vi "Is Number an IP Address.vi"(11 "UI Data in":T1={"Data Display"="", "FP Control Refs"={"Connect to Station Ref"=refnum, "Download Ref"=refnum, "Exit Button Ref"=refnum, "Start Date Refnum"=refnum, "End Date Refnum"=refnum, "Path"=refnum, "COM Port"="", "IP or Phone Ref"=refnum, "TCPIP ID"=refnum, "Reboot Refnum"=refnum, "Datafile Refnum"=refnum}, "FP Indicator Refs"={"Connected Refnum"=refnum, "Data Display Ref"=refnum, "Station ID Ref"=refnum}, "User Events"={"Stop"=refnum, "Update Display"=refnum}, "Message Queues"={"UI"=refnum, "ACQUISITION"=refnum, "PROCESSING"=refnum, "LOGGING"=refnum}, "IS IP?"=FALSE, "Downloading?"=FALSE, "DCP Version"=enum."XPert2", "Processing Loop State"=enum."Get Station  ID", "Username"=refnum, "Password"=refnum}) -> (2 "IS IP?":bool, 3 "UI Data out":T1={"Data Display"="", "FP Control Refs"={"Connect to Station Ref"=refnum, "Download Ref"=refnum, "Exit Button Ref"=refnum, "Start Date Refnum"=refnum, "End Date Refnum"=refnum, "Path"=refnum, "COM Port"="", "IP or Phone Ref"=refnum, "TCPIP ID"=refnum, "Reboot Refnum"=refnum, "Datafile Refnum"=refnum}, "FP Indicator Refs"={"Connected Refnum"=refnum, "Data Display Ref"=refnum, "Station ID Ref"=refnum}, "User Events"={"Stop"=refnum, "Update Display"=refnum}, "Message Queues"={"UI"=refnum, "ACQUISITION"=refnum, "PROCESSING"=refnum, "LOGGING"=refnum}, "IS IP?"=FALSE, "Downloading?"=FALSE, "DCP Version"=enum."XPert2", "Processing Loop State"=enum."Get Station  ID", "Username"=refnum, "Password"=refnum})   [LabVIEW 2018]
uses:
  controls/GLDL UI Data.ctl
  controls/Disconnect Control.ctl
  controls/Download Control.ctl
  controls/Exit Control.ctl
  controls/Date Control.ctl
  controls/IP Phone Number Control.ctl
  controls/Reboot Control.ctl
  controls/Connected Indicator.ctl
  controls/Output Indicator.ctl
  controls/Station ID Indicator.ctl
  Message Queue/All Message Queues.ctl
  Message Queue/Message Cluster.ctl
  controls/Processing Loop State.ctl
  Message Queue/GLDL Message Queue.lvlib
panel:
  in  "string":string
  out "IS IP? 2":bool
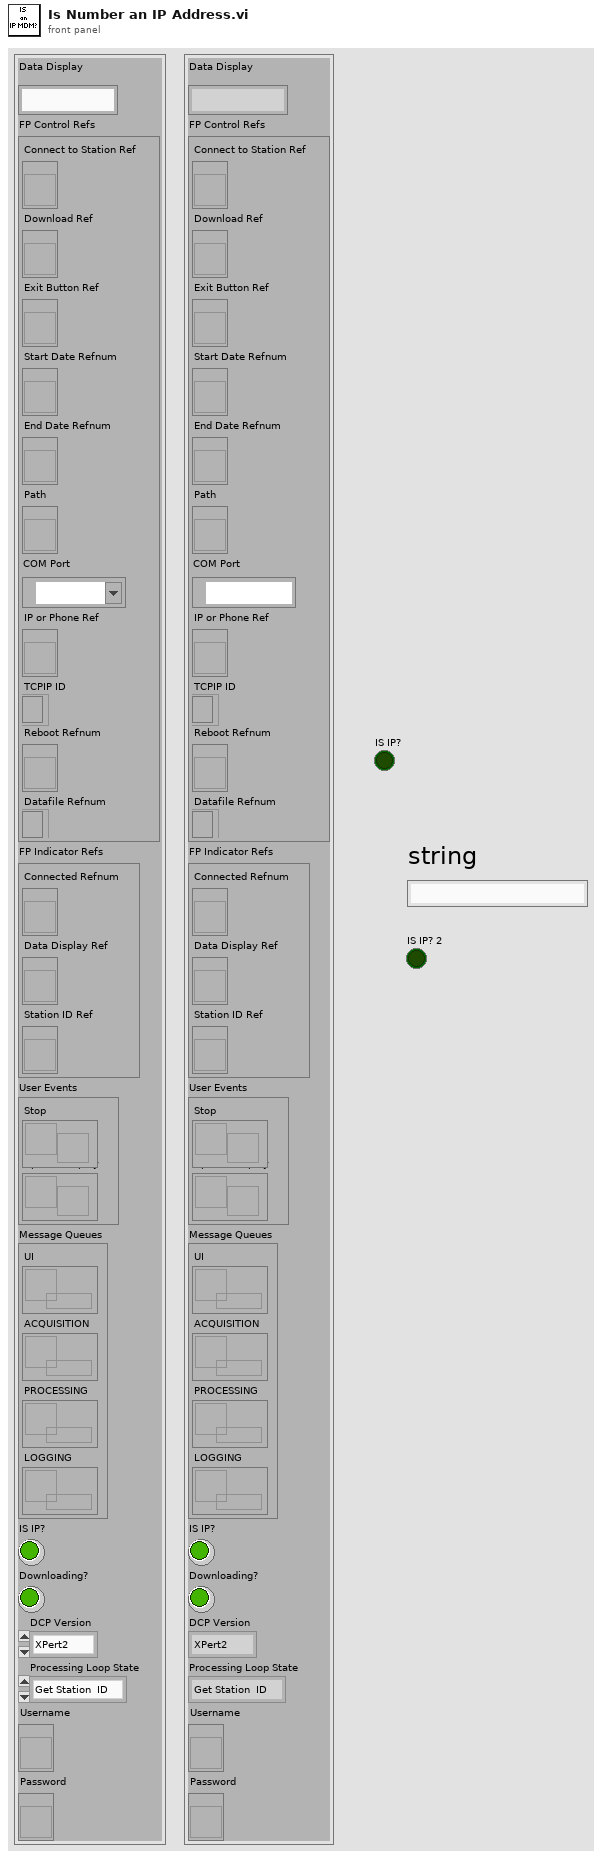
[diagram p1: front panel]
types:
  T1 = typedef "GLDL UI Data.ctl" = cluster{"Data Display":string, "FP Control Refs":cluster{"Connect to Station Ref":refnum<vi>, "Download Ref":refnum<vi>, "Exit Button Ref":refnum<vi>, "Start Date Refnum":refnum<vi>, "End Date Refnum":refnum<vi>, "Path":refnum<vi>, "COM Port":refnum<visa-resource-name>, "IP or Phone Ref":refnum<vi>, "TCPIP ID":refnum<k5>, "Reboot Refnum":refnum<vi>, "Datafile Refnum":refnum<file>}, "FP Indicator Refs":cluster{"Connected Refnum":refnum<vi>, "Data Display Ref":refnum<vi>, "Station ID Ref":refnum<vi>}, "User Events":cluster{"Stop":refnum<user-event>, "Update Display":refnum<user-event>}, "Message Queues":T2, "IS IP?":bool, "Downloading?":bool, "DCP Version":enum16{"XPert", "XPert2"}, "Processing Loop State":T3, "Username":refnum<vi>, "Password":refnum<vi>}
  T2 = typedef "GLDL Message Queue.lvlib/All Message Queues.ctl" = cluster{"UI":refnum<queue>, "ACQUISITION":refnum<queue>, "PROCESSING":refnum<queue>, "LOGGING":refnum<queue>}
  T3 = typedef "Processing Loop State.ctl" = enum16{"Get Station  ID", "Change Directory SD Card", "Change Directory Storage Card", "Downloading", "Idle in DL Directory"}
  T4 = typedef "IP Phone Number Control.ctl" = string
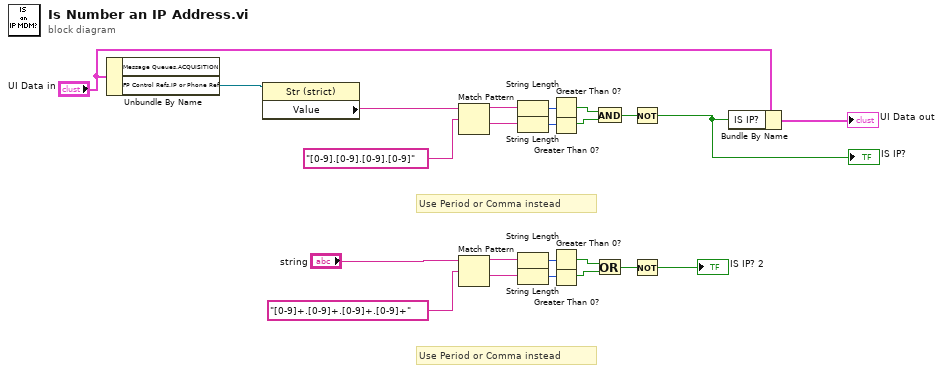
[diagram p0: block diagram]
diagram:
  # "Use Period or Comma instead"
  # "Use Period or Comma instead"
  n1 = Unbundle By Name("UI Data in") -> ("FP Control Refs.IP or Phone Ref"=w22:refnum<vi>)  [unwired: 1 out]
  n2 = property class="Str (strict)"(reference=w22) -> ("Value"=w21:T4)  [unwired: 1 in, 2 out]
  n3 = Match Pattern(string=w21, regular expression="[0-9].[0-9].[0-9].[0-9]") -> (before substring=w17:T4, after substring=w16:T4)  [unwired: 1 in, 2 out]
  n4 = Match Pattern(string="string", regular expression="[0-9]+.[0-9]+.[0-9]+.[0-9]+") -> (before substring=w5:string, after substring=w6:string)  [unwired: 1 in, 2 out]
  n5 = String Length(string=w17) -> (length=w18:i32)
  n6 = String Length(string=w16) -> (length=w13:i32)
  n7 = String Length(string=w5) -> (length=w4:i32)
  n8 = String Length(string=w6) -> (length=w9:i32)
  n9 = Greater Than 0?(x=w18) -> (x > 0?=w15:bool)
  n10 = Greater Than 0?(x=w13) -> (x > 0?=w14:bool)
  n11 = Greater Than 0?(x=w4) -> (x > 0?=w7:bool)
  n12 = Greater Than 0?(x=w9) -> (x > 0?=w8:bool)
  n13 = And(x=w15, y=w14) -> (x .and. y?=w12:bool)
  n14 = Or(x=w7, y=w8) -> (x .or. y?=w10:bool)
  n15 = Not(x=w12) -> (.not. x?=w11:bool)
  "IS IP?" <- w11
  n16 = Not(x=w10) -> (.not. x?=→"IS IP? 2":bool)
  n17 = Bundle By Name(cluster="UI Data in", "IS IP?"=w11) -> (→"UI Data out":T1)
